vi "Build Messages.vi"(8 "error in (no error)":errorcluster, 11 "Bus Controller XML Node":refnum<k20>) -> (0 "error out":errorcluster, 3 "Messages":refnum<class "Message.lvclass">[](array[class]))   [LabVIEW 2020]
doc: "Builds all the Messages defined in the BCMessages XML node. Each Message should have a unique name property."
uses:
  Frames & Messages/Message/Message.lvclass
  Frames & Messages/TypeDefs/Simplified Parameter Data Table.ctl
  Frames & Messages/TypeDefs/Scaling Information.ctl
  Frames & Messages/RT-RT Message/RT-RT Message.lvclass
  C:/Users/MattJ/Desktop/git/bci-1553-labview-api/src/RealTime/Frames & Messages/Message/Message.lvclass
  <vilib>/xml/NI_XML.lvlib
  BCI-1553 API.lvlib
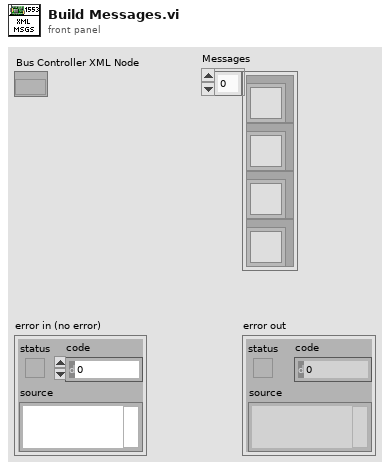
[diagram p1: front panel]
types:
  T1 = typedef "BCI-1553 API.lvlib/Simplified Parameter Data Table.ctl" = cluster{"Parameter Name":string, "Base Word":u16, "Scaling Info":T2}
  T2 = typedef "BCI-1553 API.lvlib/Scaling Information.ctl" = cluster{"Bit Offset":i32, "Bit Count":i32, "LSB Resolution":dbl, "2's Complement":bool, "Big Endian":bool, "Sign Bit":bool}
  T3 = typedef "BCI-1553 API.lvlib/Message Config.ctl" = cluster{"Time to Next Msg (4 us)":u16, "Command Config":T4, "Message Control":T9}
  T4 = typedef "BCI-1553 API.lvlib/Command Config.ctl" = cluster{"Command Type":T5, "Terminal Address":T6, "SubAddress":T7, "Word Count\\Mode Code":T8, "Command Data":u16[]}
  T5 = typedef "BCI-1553 API.lvlib/Command Type.ctl" = enum16{"Transmit", "Receive"}
  T6 = typedef "BCI-1553 API.lvlib/Command Terminal Address.ctl" = enum16{"0", "1", "2", "3", "4", "5", "6", "7", "8", "9", "10", "11", "12", "13", "14", "15", "16", "17", "18", "19", "20", "21", "22", "23", "24", "25", "26", "27", "28", "29", "30", "Broadcast"}
  T7 = typedef "BCI-1553 API.lvlib/Command SubAddress.ctl" = enum16{"Mode Code", "1", "2", "3", "4", "5", "6", "7", "8", "9", "10", "11", "12", "13", "14", "15", "16", "17", "18", "19", "20", "21", "22", "23", "24", "25", "26", "27", "28", "29", "30"}
  T8 = typedef "BCI-1553 API.lvlib/Command Word Count.ctl" = enum16{"1", "2", "3", "4", "5", "6", "7", "8", "9", "10", "11", "12", "13", "14", "15", "16", "17", "18", "19", "20", "21", "22", "23", "24", "25", "26", "27", "28", "29", "30", "31", "32"}
  T9 = typedef "BCI-1553 API.lvlib/Message Control.ctl" = cluster{"MC17 Time Sync":bool, "Error Mask":bool, "Service Request Mask":bool, "Busy Mask":bool, "SubSystem Flag Mask":bool, "Terminal Flag Mask":bool, "Reserved Mask":bool, "Retry":bool, "Bus A / !Bus B":bool, "Self-Test Loopback":bool, "Broadcast Mask":bool, "EoM Interrupt":bool, "Mode Code Format":bool, "Broadcast Format":bool, "RT-RT Format":bool}
  T10 = typedef "BCI-1553 API.lvlib/RT-RT Message Config.ctl" = cluster{"Tx Command Config":T4}
  T11 = cluster{"Parameter Name":string, "Base Word":u16, "Address":u16, "Value":u64, "Mask":u16[], "Scaling Info":cluster{"Bit Offset":i32, "Bit Count":i32, "LSB Resolution":dbl, "2's Complement":bool, "Big Endian":bool, "Sign Bit":bool}}[]
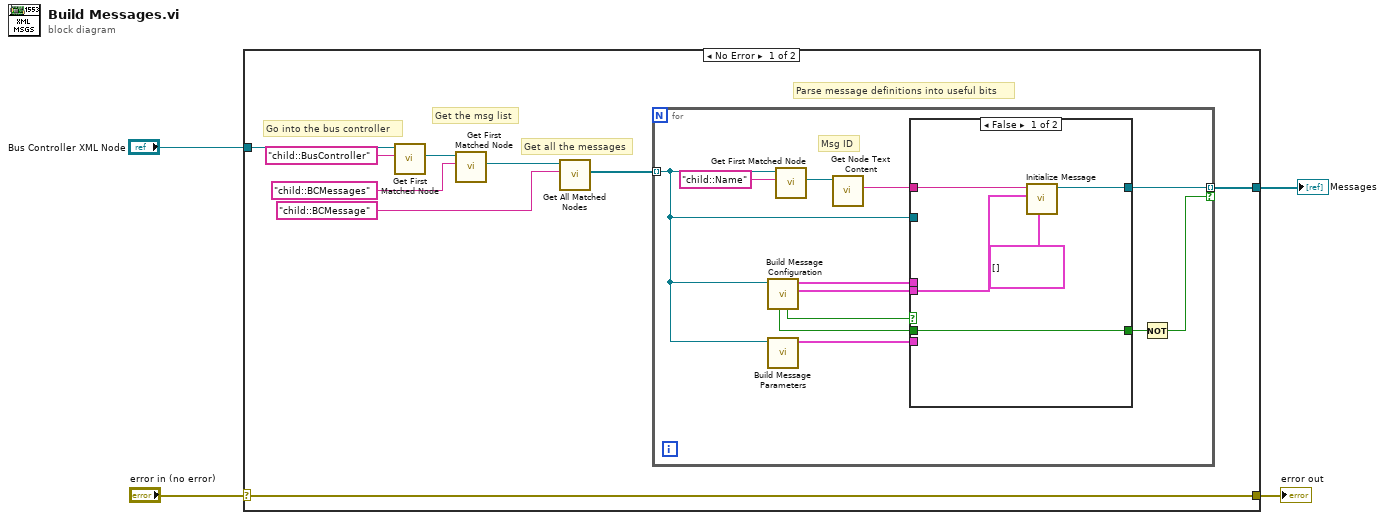
[diagram p0: block diagram]
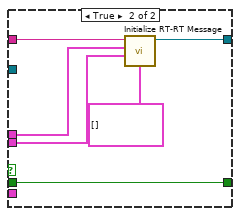
[diagram p2: hidden frame]
diagram:
  n1 = case shown="No Error" "error in (no error)" {
    selector: "error in (no error)" -> [w13 w37]
    tunnel: [w13 w37] -> w3
    tunnel: "Bus Controller XML Node" -> [w12 _]
    tunnel: [w5 _] -> w1
    frame No Error {
      # "Parse message definitions into useful bits"
      # "Get all the messages"
      # "Get the msg list"
      # "Go into the bus controller"
      n2 = call <vilib>:"Get First Matched Node.vi"("XPath expression"="child::BusController", "node in"=w12) -> ("node result"=w10:refnum<k20>)  [unwired: 7 in, 2 out]
      n3 = call <vilib>:"Get First Matched Node.vi"("XPath expression"="child::BCMessages", "node in"=w10) -> ("node result"=w8:refnum<k20>)  [unwired: 7 in, 2 out]
      n4 = call <vilib>:"Get All Matched Nodes.vi"("XPath expression"="child::BCMessage", "node in"=w8) -> ("node result array"=w6:refnum<k20>[])  [unwired: 7 in, 2 out]
      n5 = for {
        tunnel: w6 -> [w20] mode=indexing
        tunnel: [w21] -> w5 mode=indexing if=w14
        # "Msg ID"
        n6 = call "Build Message Configuration.vi"("Message XML Node"=w20) -> ("Message  Config"=w18:T3, "RT-RT Message Config"=w17:T10, "RT-RT?"=w19:bool, "Async?"=w16:bool)  [unwired: 6 in, 1 out]
        n7 = call "Build Message Parameters.vi"("Message XML Node"=w20) -> ("Parameters"=w22:T11)  [unwired: 9 in, 1 out]
        n8 = call <vilib>:"Get First Matched Node.vi"("XPath expression"="child::Name", "node in"=w20) -> ("node result"=w24:refnum<k20>)  [unwired: 7 in, 2 out]
        n9 = call <vilib>:"Get Node Text Content.vi"("node in"=w24) -> ("node text"=w23:string)  [unwired: 8 in, 2 out]
        n10 = case shown="False" w19 {
          tunnel: w23 -> [w30 w35]
          tunnel: w22 -> [_ _]
          tunnel: [w29 w36] -> w21
          tunnel: w20 -> [_ _]
          tunnel: w18 -> [w28 w34]
          tunnel: w17 -> [_ w33]
          tunnel: w16 -> [w27 w32]
          tunnel: [w27 w32] -> w15
          frame False {
            n11 = call "Initialize Message.vi"("Parameters"=T1[] [], "Message  Config"=w28, "ID"=w30) -> ("Message out"=w29:refnum<class "Message.lvclass">)  [unwired: 7 in, 1 out]
          }
          frame True {
            n12 = call "Initialize RT-RT Message.vi"("Parameters"=T1[] [], "Receive Message Config"=w34, "Transmit Message Config"=w33, "ID"=w35) -> ("RT-RT Message out"=w36:refnum<class "RT-RT Message.lvclass">)  [unwired: 6 in, 1 out]
          }
        }
        n13 = Not(x=w15) -> (.not. x?=w14:bool)
      }
    }
    frame Error {
    }
  }
  "error out" <- w3
  "Messages" <- w1
